vi "Flattened nD-Array to Flattened 1D-Array.vi"(10 "Flattened nD Array":string, 11 "nD Array Type Descriptor":i16[](array[numeric])) -> (1 "Original Dimensions":u32[](array[numeric]), 2 "Flattened 1D Array":string, 3 "1D Array Type Descriptor":i16[](array[numeric]))   [LabVIEW 2020, in "OpenDescriptor.lvlib"]
uses:
  OpenDescriptor.lvlib
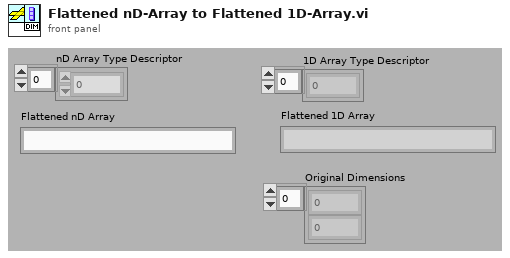
[diagram p1: front panel]
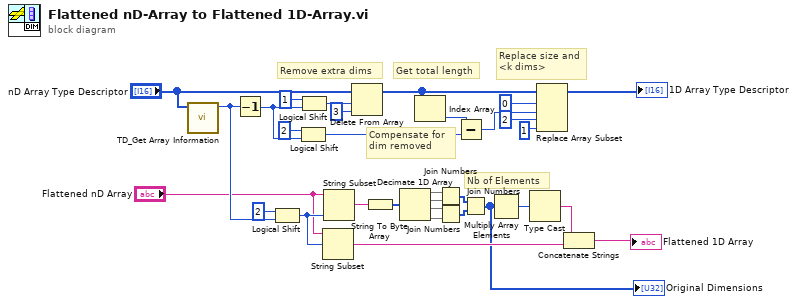
[diagram p0: block diagram]
diagram:
  # "Replace size and\n<k dims>"
  # "Compensate for\ndim removed"
  # "Get total length"
  # "Remove extra dims"
  # "Nb of Elements"
  n1 = call <vilib>:"TD_Get Array Information.vi"("Type descriptor"="nD Array Type Descriptor") -> ("Number of Dimensions"=w9:i16)  [unwired: 8 in, 2 out]
  n2 = Decrement(x=w9) -> (x-1=w20:i16)
  n3 = Logical Shift(y=i16 2, x=w9) -> (x << y=w31:i16)
  n4 = Logical Shift(y=i16 2, x=w20) -> (x << y=w21:i16)
  n5 = Logical Shift(y=i16 1, x=w20) -> (x << y=w18:i16)
  n6 = String Subset(string="Flattened nD Array", offset (0)=w31) -> (substring=w6:string)  [unwired: 1 in]
  n7 = String Subset(string="Flattened nD Array", length (rest)=w31) -> (substring=w29:string)  [unwired: 1 in]
  n8 = Delete From Array(array="nD Array Type Descriptor", length=w18, index=3) -> (array with subset deleted=w14:i16[])  [unwired: 1 out]
  n9 = String To Byte Array(string=w29) -> (unsigned byte array=w22:u8[])
  n10 = Decimate 1D Array(w22) -> (w23:u8[], w24:u8[], w25:u8[], w26:u8[])
  n11 = Index Array(array=w14) -> (element=w15:i16)  [unwired: 1 in]
  n12 = Join Numbers(hi=w23, lo=w24) -> ((hi.lo)=w28:u16[])
  n13 = Join Numbers(hi=w25, lo=w26) -> ((hi.lo)=w27:u16[])
  n14 = Subtract(x=w15, y=w21) -> (x-y=w16:i16)
  n15 = Join Numbers(hi=w28, lo=w27) -> ((hi.lo)=w1:u32[])
  "Original Dimensions" <- w1
  n16 = Multiply Array Elements(1:w1) -> (0:w8:u32)
  n17 = Type Cast(x=w8) -> (*(type *) &x=w7:string)  [unwired: 1 in]
  n18 = Replace Array Subset(array=w14, new element #1=w16, index #1=0 ("index"), new element #2=i16 1, index #2=2 ("index")) -> (→"1D Array Type Descriptor":i16[])
  n19 = Concatenate Strings(w7, w6) -> (→"Flattened 1D Array":string)
